vi "TURNTEST.vi"   [LabVIEW 2019]
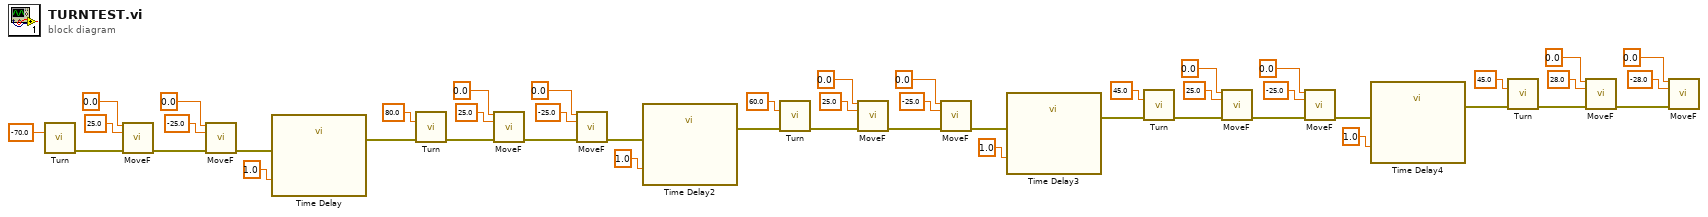
[diagram p0: block diagram]
diagram:
  n1 = call "Turn.vi"("¨¤«×"=-70.0) -> ("error out"=w2:errorcluster)  [unwired: 14 in]
  n2 = call "MoveF.vi"("X"=0.0, "Y"=25.0, "error in (no error)"=w2) -> ("error out"=w4:errorcluster)  [unwired: 12 in]
  n3 = call "MoveF.vi"("X"=0.0, "Y"=-25.0, "error in (no error)"=w4) -> ("error out"=w1:errorcluster)  [unwired: 12 in]
  n4 = call "Time Delay"("error in (no error)"=w1, "Delay Time (s)"=1.0) -> ("error out"=w44:errorcluster)  [unwired: 9 in]
  n5 = call "Turn.vi"("¨¤«×"=80.0, "error in (no error)"=w44) -> ("error out"=w9:errorcluster)  [unwired: 13 in]
  n6 = call "MoveF.vi"("X"=0.0, "Y"=25.0, "error in (no error)"=w9) -> ("error out"=w11:errorcluster)  [unwired: 12 in]
  n7 = call "MoveF.vi"("X"=0.0, "Y"=-25.0, "error in (no error)"=w11) -> ("error out"=w8:errorcluster)  [unwired: 12 in]
  n8 = call "Time Delay2"("error in (no error)"=w8, "Delay Time (s)"=1.0) -> ("error out"=w35:errorcluster)  [unwired: 9 in]
  n9 = call "Turn.vi"("¨¤«×"=60.0, "error in (no error)"=w35) -> ("error out"=w16:errorcluster)  [unwired: 13 in]
  n10 = call "MoveF.vi"("X"=0.0, "Y"=25.0, "error in (no error)"=w16) -> ("error out"=w18:errorcluster)  [unwired: 12 in]
  n11 = call "MoveF.vi"("X"=0.0, "Y"=-25.0, "error in (no error)"=w18) -> ("error out"=w15:errorcluster)  [unwired: 12 in]
  n12 = call "Time Delay3"("error in (no error)"=w15, "Delay Time (s)"=1.0) -> ("error out"=w36:errorcluster)  [unwired: 9 in]
  n13 = call "Turn.vi"("¨¤«×"=45.0, "error in (no error)"=w36) -> ("error out"=w25:errorcluster)  [unwired: 13 in]
  n14 = call "MoveF.vi"("X"=0.0, "Y"=25.0, "error in (no error)"=w25) -> ("error out"=w26:errorcluster)  [unwired: 12 in]
  n15 = call "MoveF.vi"("X"=0.0, "Y"=-25.0, "error in (no error)"=w26) -> ("error out"=w24:errorcluster)  [unwired: 12 in]
  n16 = call "Time Delay4"("error in (no error)"=w24, "Delay Time (s)"=1.0) -> ("error out"=w37:errorcluster)  [unwired: 9 in]
  n17 = call "Turn.vi"("¨¤«×"=45.0, "error in (no error)"=w37) -> ("error out"=w30:errorcluster)  [unwired: 13 in]
  n18 = call "MoveF.vi"("X"=0.0, "Y"=28.0, "error in (no error)"=w30) -> ("error out"=w31:errorcluster)  [unwired: 12 in]
  n19 = call "MoveF.vi"("X"=0.0, "Y"=-28.0, "error in (no error)"=w31) -> ()  [unwired: 12 in, 1 out]
